vi "Comprobar Temperatura Correcta.vi"(3 "error in (no error)":errorcluster, 4 "Temp.Min IN":dbl, 5 "Temp.Max  IN":dbl) -> (0 "error out":errorcluster, 1 "Temp.Min OUT":dbl, 2 "Temp.Max OUT":dbl)   [LabVIEW 2021]
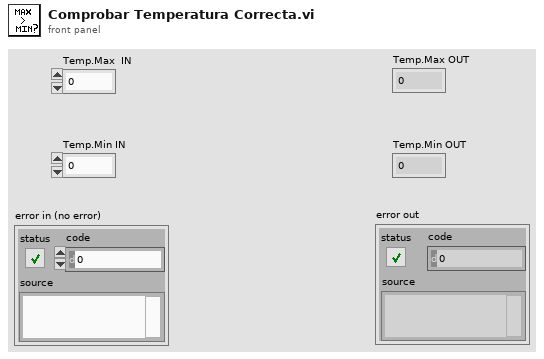
[diagram p1: front panel]
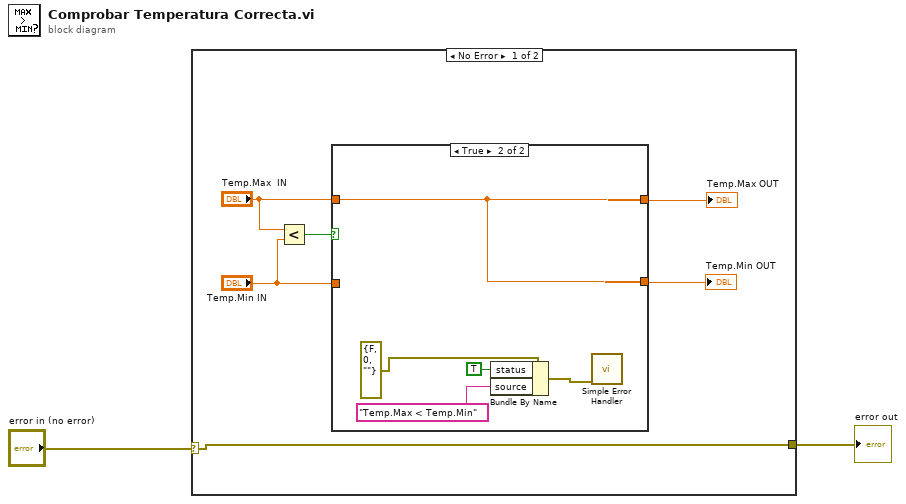
[diagram p0: block diagram]
diagram:
  n1 = case shown="No Error" "error in (no error)" {
    selector: "error in (no error)" -> [w3 w16]
    tunnel: [w3 w16] -> w1
    frame No Error {
      n2 = Less?(x="Temp.Max  IN", y="Temp.Min IN") -> (x < y?=w4:bool)
      n3 = case shown="True" w4 {
        tunnel: [w10 w15] -> w7
        tunnel: "Temp.Max  IN" -> [w10 w15]
        tunnel: [w9 w15] -> w8
        tunnel: "Temp.Min IN" -> [w9 _]
        frame False {
        }
        frame True {
          n4 = Bundle By Name(cluster=errorcluster {"status"=FALSE, "code"=0, "source"=""} ("error constant"), "status"=TRUE, "source"="Temp.Max < Temp.Min") -> (w14:errorcluster)
          n5 = call <vilib>:"Simple Error Handler.vi"("error in (no error)"=w14) -> ()  [unwired: 4 in, 5 out]
        }
      }
      "Temp.Max OUT" <- w7
      "Temp.Min OUT" <- w8
    }
    frame Error {
    }
  }
  "error out" <- w1
